vi "Update String Data.vi"(8 "error in (no error)":errorcluster, 10 "String Data":string, 11 "Status Updater in":refnum<class "Status Updater.lvclass">) -> (0 "error out":errorcluster)   [LabVIEW 2014]
uses:
  Status Updater.lvclass
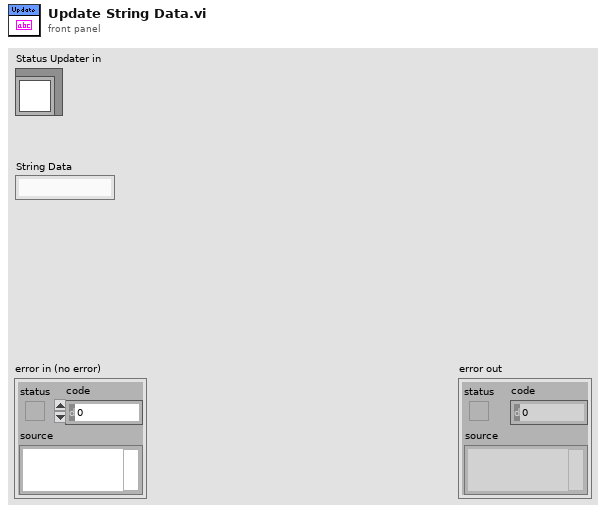
[diagram p1: front panel]
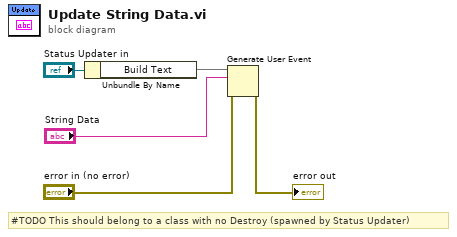
[diagram p0: block diagram]
diagram:
  # "#TODO This should belong to a class with no Destroy (spawned by Status Updater)"
  n1 = Unbundle By Name("Status Updater in") -> ("Build Text"=w4)
  n2 = Generate User Event(user event=w4, event data cluster="String Data", error in="error in (no error)") -> (error out=→"error out":errorcluster)  [unwired: 1 in, 1 out]
